vi "Read Saunders Temperature2023.vi"(3 "error in":errorcluster, 5 "Device":cluster{"GPIB #":u8, "Address":u8}={"GPIB #"=0, "Address"=28}) -> (0 "error out 2":errorcluster, 2 "Temperature":dbl format="%.2f")   [LabVIEW 2024]
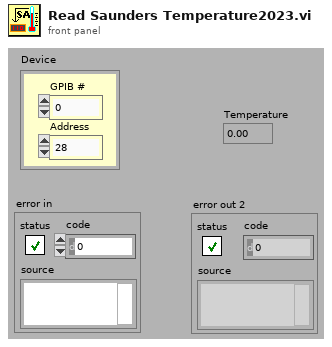
[diagram p1: front panel]
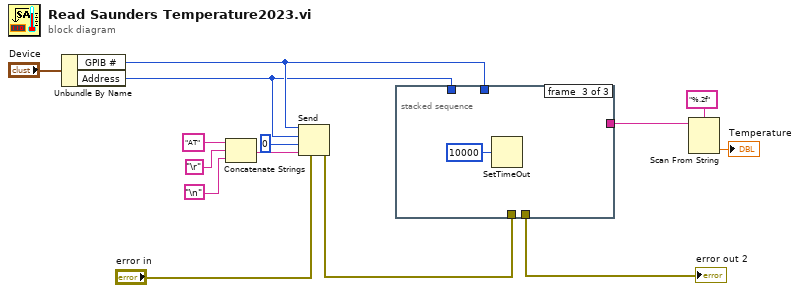
[diagram p0: block diagram]
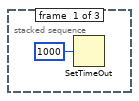
[diagram p2: hidden frame]
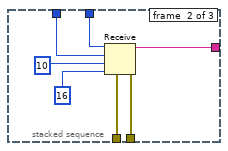
[diagram p3: hidden frame]
diagram:
  n1 = Unbundle By Name("Device") -> ("GPIB #"=w5:u8, "Address"=w4:u8)
  n2 = Concatenate Strings("AT" ("Command String"), "\r", "\n") -> (w2:string)
  n3 = Send(0:w5, 2:w4, 3:i16 0 ("mode"), 4:"error in", 5:w2) -> (8:w1:errorcluster)  [unwired: 2 out]
  n4 = stacked-sequence {
    tunnel: [_ w22 _] -> w10
    tunnel: [_ w21 _] -> w9
    tunnel: w5 -> [_ w20 _]
    tunnel: w4 -> [_ w19 _]
    tunnel: w1 -> [_ w16 _]
    frame #0 {
      n5 = SetTimeOut(1:1000 ("new timeout (10000)")) -> ()  [unwired: 1 out]
    }
    frame #1 {
      n6 = Receive(4:w16, 6:16 ("count"), 7:i16 10 ("mode"), 8:w19, 9:w20) -> (0:w22:errorcluster, 3:w21:string)  [unwired: 2 out]
    }
    frame #2 {
      n7 = SetTimeOut(1:10000 ("new timeout (10000)")) -> ()  [unwired: 1 out]
    }
  }
  "error out 2" <- w10
  n8 = Scan From String(format string="%.2f", input string=w9) -> (output 1=→"Temperature":dbl)  [unwired: 3 in, 3 out]
